vi "DMR_GetImageRequestBufferImageData8bit.vi"(0 "driver handle IN":u32, 1 "request number IN":u32, 2 "bytes per pixel IN":u32, 4 "X-offset":u32, 5 "Y-offset":u32, 7 "height":u32, 9 "width":u32) -> (14 "driver handle OUT":u32, 15 "request number OUT":u32, 17 "image OUT":u8[][](array[numeric]), 19 "error code OUT":i32)   [LabVIEW 2014]
uses:
  C:/Users/temp/Desktop/labview UHR-Fleezers instrument control/MATRIX VISION/LabVIEW_Acquire.dll
panel:
  # "INPUT"
  # "OUTPUT"
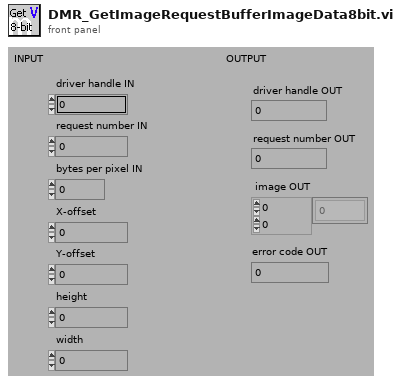
[diagram p1: front panel]
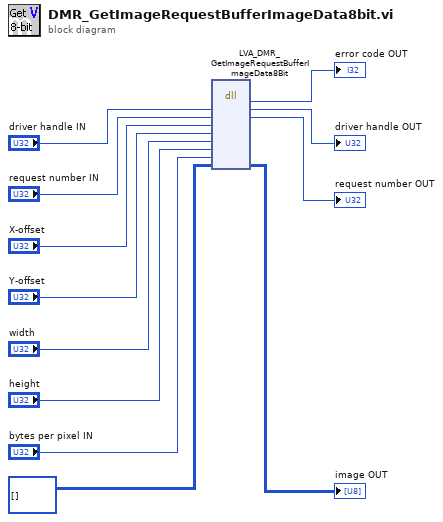
[diagram p0: block diagram]
diagram:
  n1 = dll-call lib="C:/Users/temp/Desktop/labview UHR-Fleezers instrument control/MATRIX VISION/LabVIEW_Acquire.dll" fn="LVA_DMR_GetImageRequestBufferImageData8Bit"("hDrv"="driver handle IN", "requestNr"="request number IN", "XOffset"="X-offset", "YOffset"="Y-offset", "width"="width", "height"="height", "bytespp"="bytes per pixel IN", "ppImageData"=u8[][] [] ("pImageData")) -> (→"error code OUT":i32, "hDrv"=→"driver handle OUT":i32, "requestNr"=→"request number OUT":i32, "ppImageData"=→"image OUT":i8[][])  [unwired: 8 in, 2 out]
